vi "FITS_CreateFile_Simple.vi"(8 "error in":errorcluster, 10 "filename":string) -> (0 "error out":errorcluster, 2 "result":i32, 3 "fd":u64)   [LabVIEW 2016]
uses:
  usr/local/lib/libfits.so
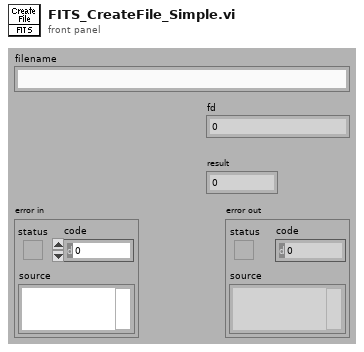
[diagram p1: front panel]
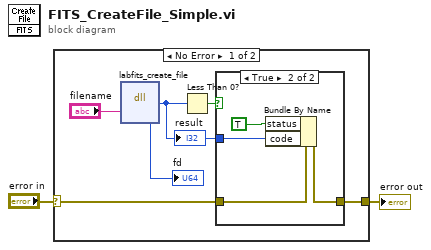
[diagram p0: block diagram]
diagram:
  n1 = case shown="No Error" "error in" {
    selector: "error in" -> [w6 w14]
    tunnel: [w5 w14] -> w1
    frame No Error {
      n2 = dll-call lib="usr/local/lib/libfits.so" fn="labfits_create_file"("filename"="filename") -> ("return type"=w4:i32, "fd"=→"fd":u64)  [unwired: 4 in, 3 out]
      "result" <- w4
      n3 = Less Than 0?(x=w4) -> (x < 0?=w7:bool)
      n4 = case shown="True" w7 {
        tunnel: w6 -> [w9 w11]
        tunnel: [w9 w10] -> w5
        tunnel: w4 -> [_ w12]
        frame False {
        }
        frame True {
          n5 = Bundle By Name(cluster=w11, "status"=TRUE, "code"=w12) -> (w10:errorcluster)
        }
      }
    }
    frame Error {
    }
  }
  "error out" <- w1
